vi "Solution part 1.vi"() -> ()   [LabVIEW 2020]
uses:
  <vilib>/Utility/error.llb/Error Cluster From Error Code.vi
  <vilib>/ErrorRing/Error Ring.xnode
panel:
  out "error out":errorcluster
  out "result":i64
  in  "data?":bool
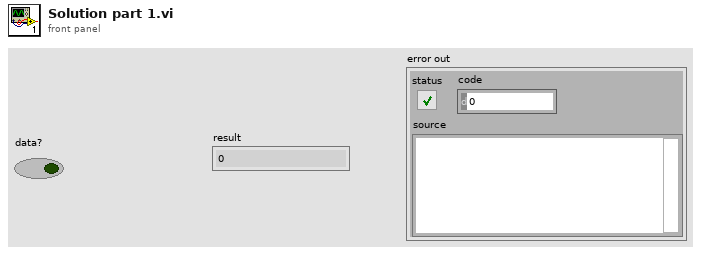
[diagram p1: front panel]
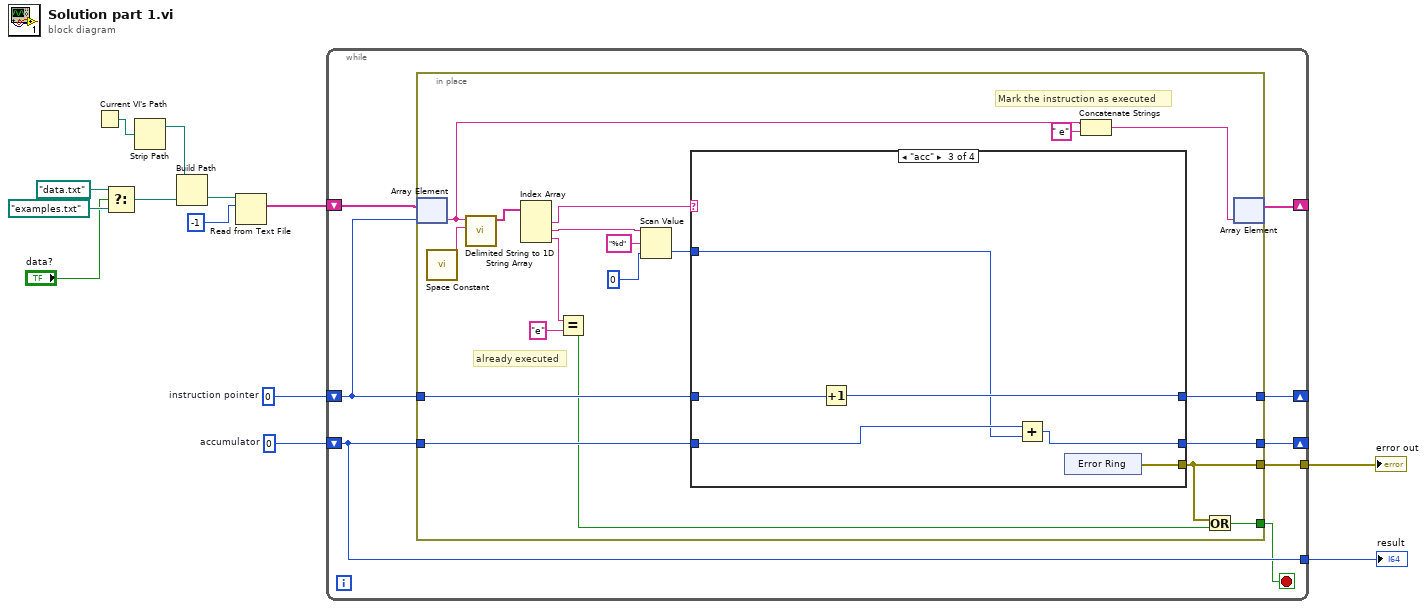
[diagram p0: block diagram]
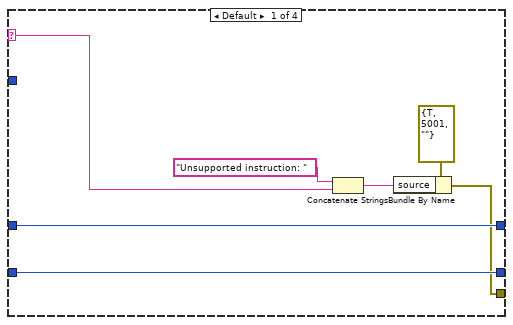
[diagram p2: hidden frame]
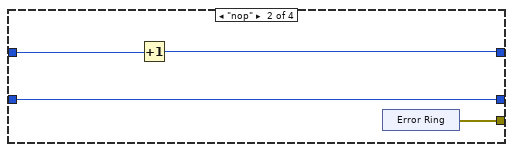
[diagram p3: hidden frame]
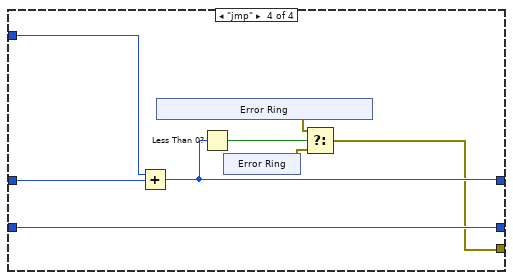
[diagram p4: hidden frame]
diagram:
  w2 = i64 0  # instruction pointer
  w4 = i64 0  # accumulator
  n1 = Current VI's Path() -> (path=w9:path)
  n2 = Select(t=path "data.txt", s="data?", f=path "examples.txt") -> (s? t:f=w10:path)
  n3 = Strip Path(path=w9) -> (stripped path=w8:path)  [unwired: 1 out]
  n4 = Build Path(base path=w8, name or relative path=w10) -> (appended path=w7:path)
  n5 = Read from Text File(file (use dialog)=w7, count=-1) -> (text=w5:string[])  [unwired: 2 in, 3 out]
  n6 = while {
    shift-right: [w20] -> _
    shift-left: w4 -> [w21]
    tunnel: [w21] -> w3
    shift-right: [w19] -> _
    shift-left: w2 -> [w16]
    shift-right: [w14] -> _
    shift-left: w5 -> [w17]
    tunnel: [w15] -> w1
    stop <- w18 stop-if-true
    n7 = in-place {
      in-place-border: w21 -> [w40]
      in-place-border: [w39] -> w20
      in-place-border: [w38] -> w19
      in-place-border: w16 -> [w37]
      in-place-border: [w29] -> w18
      in-place-border: [w28] -> w15
      # "Mark the instruction as executed"
      # "already executed"
      n8 = in-place-array #1(w17, w16) -> (w27:string)
      n9 = call <vilib>:"Space Constant.vi"() -> ("String"=w33:string)
      n10 = call <vilib>:"Delimited String to 1D String Array.vi"("delimiter"=w33, "delimited string"=w27) -> ("string array"=w32:string[])  [unwired: 9 in]
      n11 = Index Array(array=w32) -> (element #1=w31:string, element #2=w30:string, element #3=w24:string)  [unwired: 3 in]
      n12 = Equal?(x=w24, y="e") -> (x = y?=w22:bool)
      n13 = Scan Value(string=w30, format string="%d", default (0 dbl)=i64 0) -> (value=w35:i64)  [unwired: 1 out]
      n14 = case shown="\"acc\"" w31 {
        selector: w31 -> [w42 _ _ _]
        tunnel: w40 -> [w47 w51 w58 w67]
        tunnel: [w47 w51 w54 w67] -> w39
        tunnel: w37 -> [w46 w50 w57 w66]
        tunnel: [w46 w49 w56 w64] -> w38
        tunnel: w35 -> [_ _ w53 w65]
        tunnel: [w41 w48 w55 w60] -> w28
        frame Default {
          n15 = Concatenate Strings("Unsupported instruction: " ("source 2"), w42) -> (w44:string)
          n16 = Bundle By Name(cluster=errorcluster {"status"=TRUE, "code"=5001, "source"=""} ("error constant"), "source"=w44) -> (w41:errorcluster)
        }
        frame "nop" {
          n17 = Increment(x=w50) -> (x+1=w49:i64)
          n18 = xnode "Error Ring"() -> ("error out"=w48:errorcluster)
        }
        frame "acc" {
          n19 = Increment(x=w57) -> (x+1=w56:i64)
          n20 = Add(x=w58, y=w53) -> (x+y=w54:i64)
          n21 = xnode "Error Ring"() -> ("error out"=w55:errorcluster)
        }
        frame "jmp" {
          n22 = Add(x=w65, y=w66) -> (x+y=w64:i64)
          n23 = xnode "Error Ring"() -> ("error out"=w61:errorcluster)
          n24 = Less Than 0?(x=w64) -> (x < 0?=w63:bool)
          n25 = xnode "Error Ring"() -> ("error out"=w62:errorcluster)
          n26 = Select(t=w61, s=w63, f=w62) -> (s? t:f=w60:errorcluster)
        }
      }
      n27 = Concatenate Strings(w27, " e" ("string")) -> (w25:string)
      n28 = Or(x=w28, y=w22) -> (x .or. y?=w29:bool)
      n29 = in-place-array #1(w25) -> (w14:string[])  [unwired: 1 out]
    }
  }
  "result" <- w3
  "error out" <- w1
